vi "Get Shutter Min Times.vi"(8 "error in (no error)":errorcluster, 10 "minopeningtime":i32, 11 "minclosingtime":i32) -> (0 "error out":errorcluster, 1 "function return":u32, 2 "minopeningtime out":i32, 3 "minclosingtime out":i32)   [LabVIEW 2014, in "atmcd32d.lvlib"]
doc: "unsigned int WINAPI GetShutterMinTimes(int * minclosingtime, int * minopeningtime);"
uses:
  atmcd32d.lvlib
  atmcd32d.dll
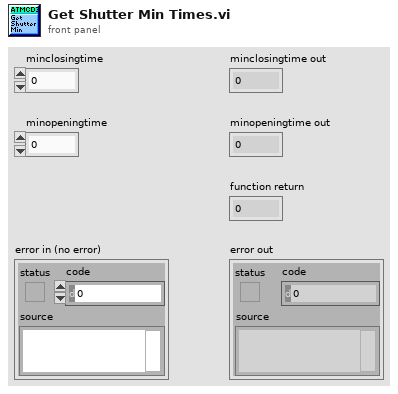
[diagram p1: front panel]
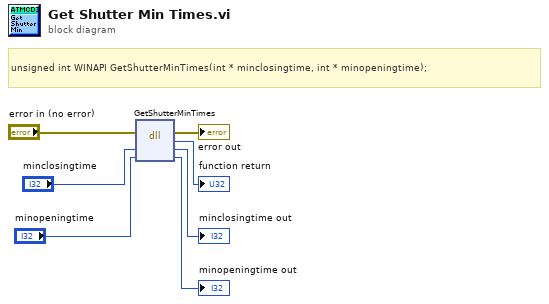
[diagram p0: block diagram]
diagram:
  # "unsigned int WINAPI GetShutterMinTimes(int * minclosingtime, int * minopeningtime);"
  n1 = dll-call lib="C:/Users/Bakir/Documents/Lambda2-Testing/lib/Andorlib/atmcd32d.*" fn="GetShutterMinTimes"(error in="error in (no error)", "minclosingtime"="minclosingtime", "minopeningtime"="minopeningtime") -> (error out=→"error out":errorcluster, →"function return":u32, "minclosingtime"=→"minclosingtime out":i32, "minopeningtime"=→"minopeningtime out":i32)  [unwired: 2 in, 1 out]
